vi "Prova TuroVibrazioni.vi"() -> ()   [LabVIEW 2016]
uses:
  <vilib>/addons/_NISVFA/_Shared subVIs/Controls/svc_Channel Info.ctl
  <vilib>/addons/_NISVFA/_Shared subVIs/Controls/svc_Engineering Units Text Ring.ctl
  <vilib>/addons/_NISVFA/_Shared subVIs/Controls/svc_Weighting Filter Text Ring.ctl
  <vilib>/DAQmx/read.llb/DAQmx Read (Analog Wfm 1Chan NSamp).vi
  <vilib>/addons/Sound and Vibration/svt_Calibration/SVL Scale Voltage to EU (1 Ch).vi
  <vilib>/addons/_NISVFA/_Shared subVIs/Common/svc_Set SV Channel Info.vi
  <vilib>/addons/_NISVFA/_Shared subVIs/Common/svc_Set SV Channel Info (variant).vi
  <vilib>/addons/_NISVFA/_Shared subVIs/Common/SVL Set dB Reference (variant).vi
  <vilib>/DAQmx/create/channels.llb/DAQmx Create Channel (AI-Acceleration-Accelerometer).vi
  <vilib>/DAQmx/configure/timing.llb/DAQmx Timing (Sample Clock).vi
  <vilib>/DAQmx/miscellaneous.llb/DAQmx Fill In Error Info.vi
  <vilib>/addons/Sound and Vibration/Order Analysis/Referece Data Processing/OAT IIR Preprocess Filter (1 Channel).vi
  <vilib>/addons/_NISVFA/_Shared subVIs/Common/svc_Engineering Units to Unit Label.vi
  <vilib>/addons/_NISVFA/_Shared subVIs/Common/svc_Compute Scale Factor to Convert V to EU.vi
  <vilib>/addons/_NISVFA/_Shared subVIs/Common/svc_Set dB ref if Pascal.vi
  <vilib>/addons/_NISVFA/_Shared subVIs/Common/svc_Caller VI Returned in Error Source.vi
  <vilib>/addons/Sound and Vibration/svt_Integration/SVL Integration (N Ch).vi
  <vilib>/measure/madcrms.llb/Basic Averaged DC-RMS for 1 Chan.vi
  <vilib>/addons/Sound and Vibration/svt_Integration/SoundVib_Integration.lvlib
  <vilib>/measure/NI_MAPro.lvlib
  <vilib>/addons/Sound and Vibration/svt_Calibration/SoundVib_Calibration.lvlib
  <vilib>/addons/Sound and Vibration/Order Analysis/Referece Data Processing/SoundVib_RefDataProcess.lvlib
panel:
  in  "freq specs [Hz]":T1={"low cutoff freq"=1.0, "high cutoff freq"=1.0} {"high cutoff freq" format="%#.2f"; "low cutoff freq" format="%#.4f"}
  in  "measurement info":T2={"uncertainty"=0.0, "Warning"=FALSE, "comments"="reserved for future use"} {"uncertainty" format="%0.2p"}
  out "DC value":dbl format="%0.2p"
  in  "highpass cutoff frequency":dbl=1.0 format="%.2f"
  in  "number of samples per channel":i32=-1
  in  "channel info":T3={"sensor sensitivity [mV/EU]"=1000.0, "engineering units"=2, "dB reference [EU]"=2e-05, "custom label"="EU", "weighting filter"=0, "pregain [dB]"=0.0} {"pregain [dB]" format="%.2f"; "weighting filter" items=["Linear", "A-weighting", "B-weighting", "C-weighting", "ITU-R 468-4", "Dolby", "CCITT", "C-message", "Wb", "Wc", "Wd", "We", "Wf", "Wh", "Wj", "Wk", "Wm", "AES17 20 kHz lowpass", "AES17 40 kHz lowpass", "AES17 20 kHz highpass", "AES17 40 kHz highpass"]; "dB reference [EU]" format="%^.1e"; "engineering units" items=["custom..."=0, "V"=1, "A"=21, "Pa"=2, "N"=20, "g"=3, "m/s^2"=4, "m/s"=5, "m"=6, "mm/s"=12, "mm"=13, "micron/s"=14, "micron"=15, "in/s^2"=7, "in/s"=8, "in"=9, "mil/s"=10, "mil"=11, "rad/s^2"=16, "rad/s"=17, "rad"=18, "deg/s^2"=26, "deg/s"=27, "deg"=28, "RPM"=22, "cycle/s^2"=23, "Hz"=24, "cycle"=25, "strain"=19]; "sensor sensitivity [mV/EU]" format="%.2f"}
  in  "window":T6(ring)
  in  "averaging type":enum16{"Linear", "Exponential"}(ring)
  out "RMS value":dbl format="%.4f"
  out "data":waveform(dbl)
  out "error out":errorcluster
  in  "rate":dbl=1000.0 format="%0.2f"
  in  "physical channels":tag
  in  "quit":bool
  out "Acceleration":waveform(dbl)[](graph)
  out "integrated signal":waveform(dbl)[](graph) caption="Velocity"
  out "XY Plot":cluster{"Y":dbl[], "Y":dbl[]}(graph)
  in  "velocity - displacement":T7(ring)=enum."double integration"
  in  "reset filter":bool
  in  "length units":i32(ring)=2 items=["no change"=-1, "m"=0, "mm"=2, "microns"=3, "in"=1, "mils"=5]
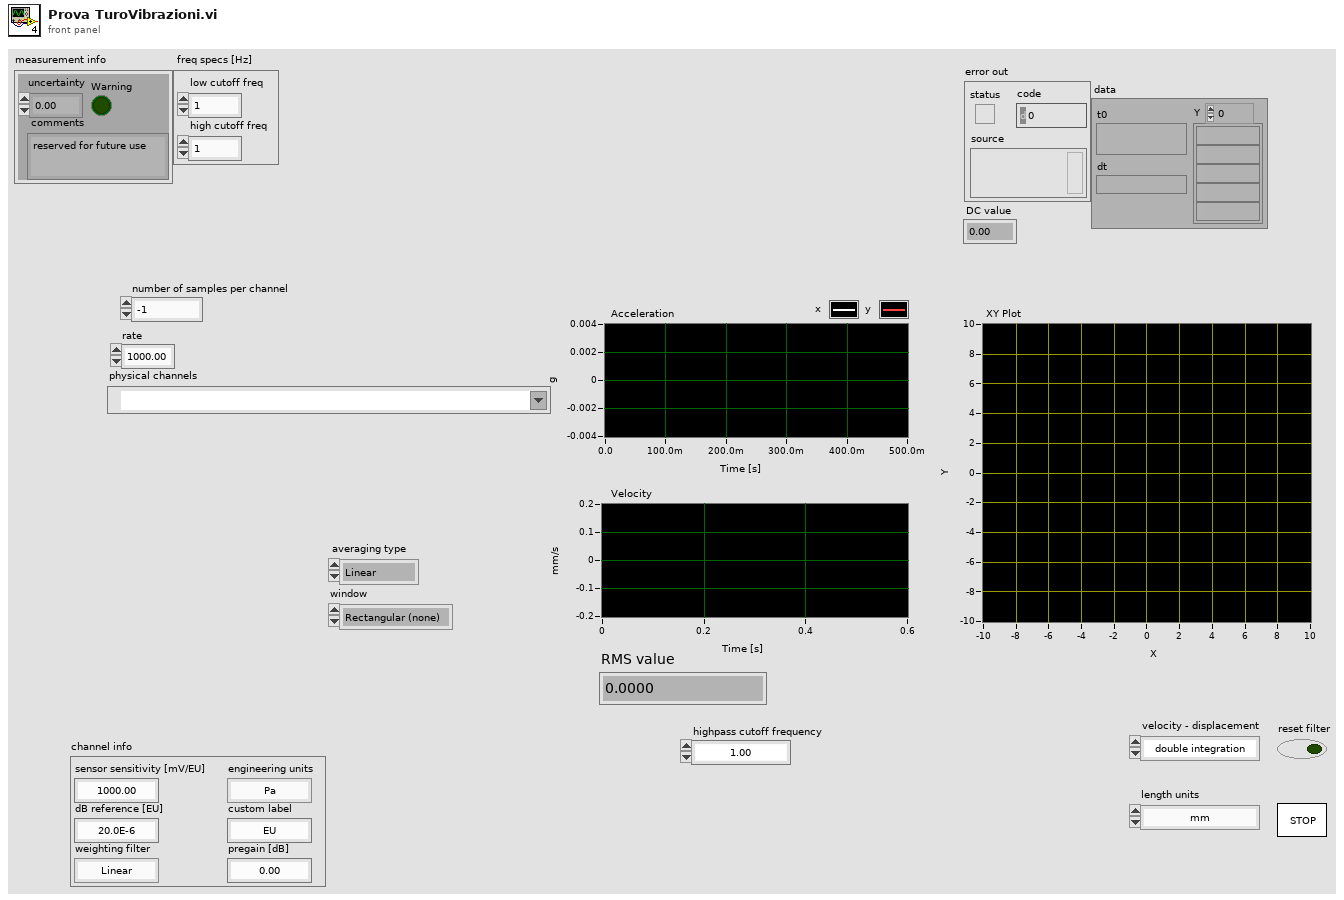
[diagram p1: front panel]
types:
  T1 = cluster{"low cutoff freq":dbl, "high cutoff freq":dbl}
  T2 = cluster{"uncertainty":dbl, "Warning":bool, "comments":string}
  T3 = typedef "svc_Channel Info.ctl" = cluster{"sensor sensitivity [mV/EU]":dbl, "engineering units":T4, "dB reference [EU]":dbl, "custom label":string, "weighting filter":T5, "pregain [dB]":dbl}
  T4 = typedef "svc_Engineering Units Text Ring.ctl" = u16
  T5 = typedef "svc_Weighting Filter Text Ring.ctl" = u16
  T6 = enum16{"Rectangular (none)", "Hanning", "Low side lobe"}
  T7 = enum16{"single integration", "double integration"}
  T8 = enum32{"Lowpass", "Highpass", "Bandpass", "Bandstop"}
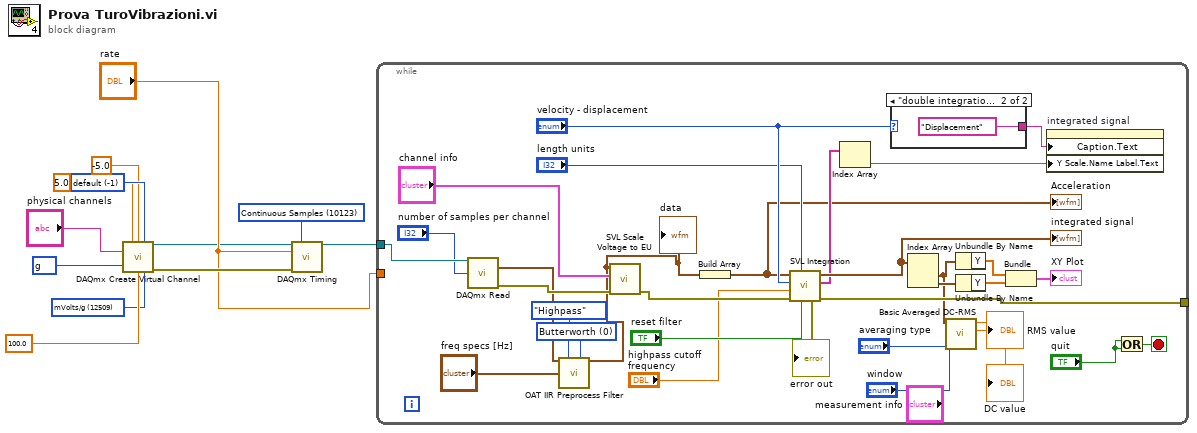
[diagram p0: block diagram]
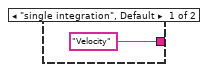
[diagram p2: hidden frame]
diagram:
  w5 = 12509 items=["mVolts/g"=12509, "Volts/g"=12510] ("sensitivity units")
  w7 = 10186 items=["g"=10186, "m/s^2"=12470, "in/s^2"=12471, "From Custom Scale"=10065] ("units")
  w8 = -1 items=["default"=-1, "RSE"=10083, "NRSE"=10078, "Differential"=10106, "Pseudodifferential"=12529] ("input terminal configuration")
  w11 = 10123 items=["Finite Samples"=10178, "Continuous Samples"=10123, "Hardware Timed Single Point"=12522] ("sample mode")
  n1 = call-poly <vilib>:"DAQmx Create Virtual Channel.vi"("maximum value"=5.0, "minimum value"=-5.0, "input terminal configuration"=w8, "physical channels"="physical channels", "units"=w7, "sensitivity"=100.0, "sensitivity units"=w5) -> ("task out"=w1:refnum<k21>, "error out"=w10:errorcluster)  [unwired: 7 in]
  n2 = call-poly <vilib>:"DAQmx Timing.vi"("task/channels in"=w1, "sample mode"=w11, "rate"="rate", "error in"=w10) -> ("task out"=w2:refnum<k21>)  [unwired: 10 in, 1 out]
  n3 = while {
    tunnel: [w34] -> _
    tunnel: w2 -> [w31]
    tunnel: "rate" -> [_]
    stop <- w43 stop-if-true
    w15 = u16 0 items=["Butterworth", "Chebyshev", "Inverse Chebyshev", "Elliptic"] ("design method")
    n4 = call-poly <vilib>:"DAQmx Read.vi"("task/channels in"=w31, "number of samples per channel"="number of samples per channel") -> ("data"=w14:waveform(dbl), "error out"=w24:errorcluster)  [unwired: 11 in, 1 out]
    n5 = call-poly <vilib>:"OAT IIR Preprocess Filter.vi"("scaled signal [EU]"=w14, "filter type"=T8."Highpass", "design method"=w15, "freq specs [Hz]"="freq specs [Hz]") -> ("filtered scaled signal [EU]"=w13:waveform(dbl))  [unwired: 10 in, 1 out]
    "data" <- w13
    n6 = call-poly <vilib>:"SVL Scale Voltage to EU.vi"("error in (no error)"=w24, "channel info"="channel info", "signal [V]"=w13) -> ("error out"=w23:errorcluster)  [unwired: 6 in, 2 out]
    n7 = Build Array(w13) -> (w29:waveform(dbl)[])
    "Acceleration" <- w29
    n8 = call-poly <vilib>:"SVL Integration.vi"("reset filter (F)"="reset filter", "length units"="length units", "error in (no error)"=w23, "highpass cutoff frequency"="highpass cutoff frequency", "integration type"="velocity - displacement", "scaled signals [EU]"=w29) -> ("error out"=w34:errorcluster, "unit labels"=w30:string[], "integrated signals"=w35:waveform(dbl)[])  [unwired: 3 in]
    "integrated signal" <- w35
    "error out" <- w34
    n9 = Index Array(array=w30) -> (element=w39:string)  [unwired: 1 in]
    n10 = case shown="\"double integration\"" "velocity - displacement" {
      tunnel: ["Velocity" ("Label.Text") "Displacement" ("Label.Text")] -> w40
      frame "single integration", Default {
      }
      frame "double integration" {
      }
    }
    n11 = Index Array(array=w35) -> (element #1=w27:waveform(dbl), element #2=w32:waveform(dbl))  [unwired: 2 in]
    n12 = call-poly <vilib>:"Basic Averaged DC-RMS.vi"("window"="window", "averaging type"="averaging type", "signal in"=w27) -> ("RMS value"=→"RMS value":dbl, "DC value"=→"DC value":dbl)  [unwired: 5 in, 2 out]
    n13 = Unbundle By Name(w27) -> ("Y"=w36:dbl[])
    n14 = Unbundle By Name(w32) -> ("Y"=w37:dbl[])
    n15 = Bundle("Y"=w36, "Y"=w37) -> (→"XY Plot":cluster{"Y":dbl[], "Y":dbl[]})  [unwired: 1 in]
    n16 = property on="integrated signal" class="WFGraph (strict)"("Caption.Text"=w40, "Y Scale.Name Label.Text"=w39) -> ()  [unwired: 2 in, 2 out]
    n17 = Or(x="quit", y="quit") -> (x .or. y?=w43:bool)
  }
